vi "Robot Global Data.vi"() -> ()   [LabVIEW 2014]
doc: "This global VI can contain as many global variables as you need. Place a control on the panel, give it a good name. To read or write to it from a VI, drag the icon to the diagram of that VI. You can also drag from the project. Click on the node to change which global you access. You shouldn't have multiple locations writing to a global or it will cause a race-condition."
uses:
  <vilib>/Rock Robotics/WPI/Camera/WPI_CameraImageSize.ctl
  <vilib>/Rock Robotics/WPI/DriverStation/WPI_DriverStationRobotMode2.ctl
panel:
  in  "encLiftRate":dbl
  out "inLoop":bool
  in  "leftRate":dbl
  in  "rightRate":dbl
  in  "rightEncoderDistance":dbl
  in  "leftEncoderDistance":dbl
  out "toteLift":bool
  out "liftMot":bool
  out "changeState":bool
  in  "desiredState":enum16{"binUp", "toteUp", "down"}(ring)
  in  "currentState":enum16{"binUp", "toteUp", "down"}(ring)
  in  "Encoder Spins per Revolution":dbl
  in  "Gear State":enum16{"Low Gear", "High Gear"}(ring)
  out "clampsBack":bool
  out "clampsFor":bool
  out "elevatorFor":bool
  out "elevatorBack":bool
  in  "Intake State":enum16{"neutral", "rotate", "intake", "eject"}(ring)
  out "intakeBack":bool
  out "intakeFor":bool
  out "secButton2":bool
  out "secButton6":bool
  out "secButton5":bool
  in  "lift":dbl
  in  "right":dbl
  in  "left":dbl
  out "rightButton3":bool
  out "rightButton2":bool
  in  "Robot Mode":T1
  in  "image size":T2=enum."320x240"
  in  "Enable Vision":bool
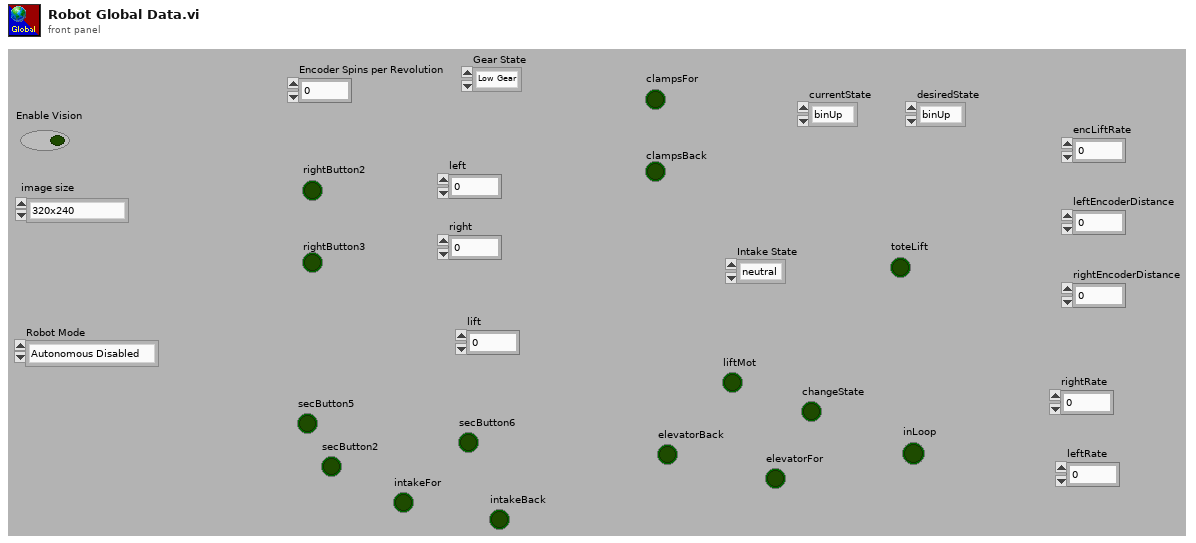
[diagram p1: front panel]
types:
  T1 = typedef "WPI_DriverStationRobotMode2.ctl" = enum16{"Autonomous Disabled", "Autonomous Enabled", "Teleop Disabled", "Teleop Enabled", "Disconnected", "Finish", "Test Disabled", "Test Enabled", "Emergency Stopped"}
  T2 = typedef "WPI_CameraImageSize.ctl" = enum16{"640x480", "320x240", "160x120", "Custom"}
diagram:
